vi "Set Speed.vi"(8 "error in (no error)":errorcluster, 10 "Speed":dbl, 11 "Motor in":refnum<class "Motor.lvclass">) -> (0 "error out":errorcluster, 3 "Motor out":refnum<class "Motor.lvclass">)   [LabVIEW 2026, in "Motor.lvlib" / "Motor.lvclass"]
uses:
  Motor.lvclass
  Motor.lvclass/Motor.ctl
  CTI-Grove/Examples/Sourcecode/cti-drivers-lv-visa-simple/Examples/Driver/CTIPicoVISA.lvlib
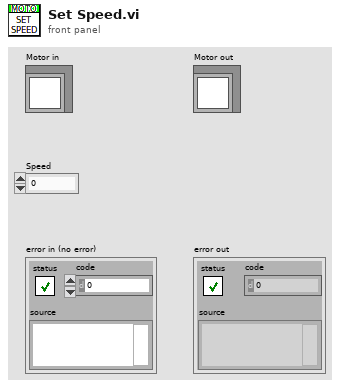
[diagram p1: front panel]
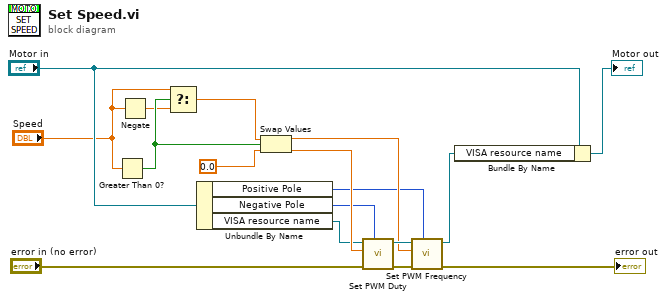
[diagram p0: block diagram]
diagram:
  n1 = Greater Than 0?(x="Speed") -> (x > 0?=w4:bool)
  n2 = Negate(x="Speed") -> (-x=w2:dbl)
  n3 = Select(t="Speed", s=w4, f=w2) -> (s? t:f=w3:dbl)
  n4 = Unbundle By Name("Motor in") -> ("Positive Pole"=w11:i32, "Negative Pole"=w13:i32, "VISA resource name"=w12:refnum<visa-resource-name>)
  n5 = Swap Values(12:w3, 13:w4, 14:0.0 ("Speed")) -> (1:w15:dbl, 3:w16:dbl)
  n6 = call "Set PWM Duty.vi"("GPIO"=w13, "error in (no error)"="error in (no error)", "Duty % (0-1)"=w16, "VISA resource name in"=w12) -> ("error out"=w7:errorcluster, "VISA resource name"=w17:refnum<visa-resource-name>)  [unwired: 6 in]
  n7 = call "Set PWM Frequency.vi"("GPIO"=w11, "error in (no error)"=w7, "Freq Hz"=w15, "VISA resource name in"=w17) -> ("error out"=→"error out":errorcluster, "VISA resource name"=w9:refnum<visa-resource-name>)  [unwired: 6 in]
  n8 = Bundle By Name(cluster="Motor in", "VISA resource name"=w9) -> (→"Motor out":refnum<class "Motor.lvclass">)
